vi "Filter_String_Parser.vi"(11 "Filter String":string="Protocol == UDP AND Length > 0.7 OR Source == 192.168.1.1") -> (1 "Comparators":T1(array[cluster]), 3 "Boolean Connectors":string[](array[string]))   [LabVIEW 2025, in "Table_Filtering.lvlib"]
uses:
  Table_Filtering.lvlib
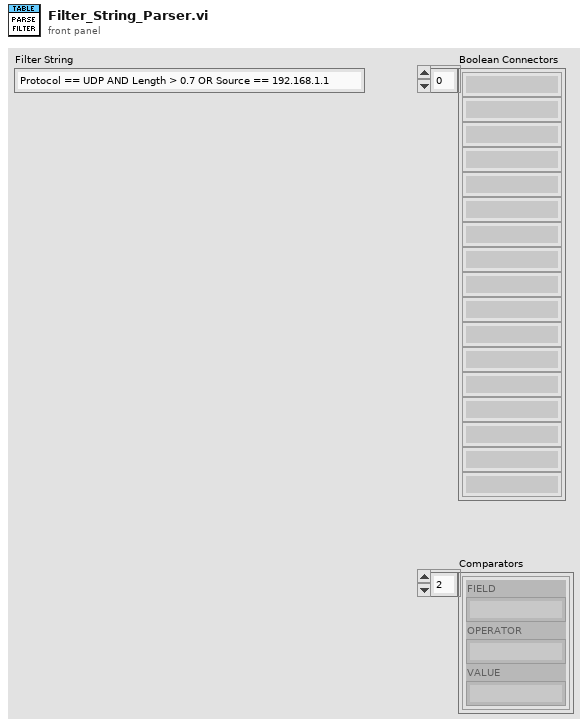
[diagram p1: front panel]
types:
  T1 = cluster{"FIELD":string, "OPERATOR":string, "VALUE":string}[]
  T2 = cluster{"FIELD":string, "OPERATOR":string, "VALUE":string}
  T3 = enum16{"Packet Number", "Timestamp", "Source", "Destination", "Protocol", "Length", "Data"}
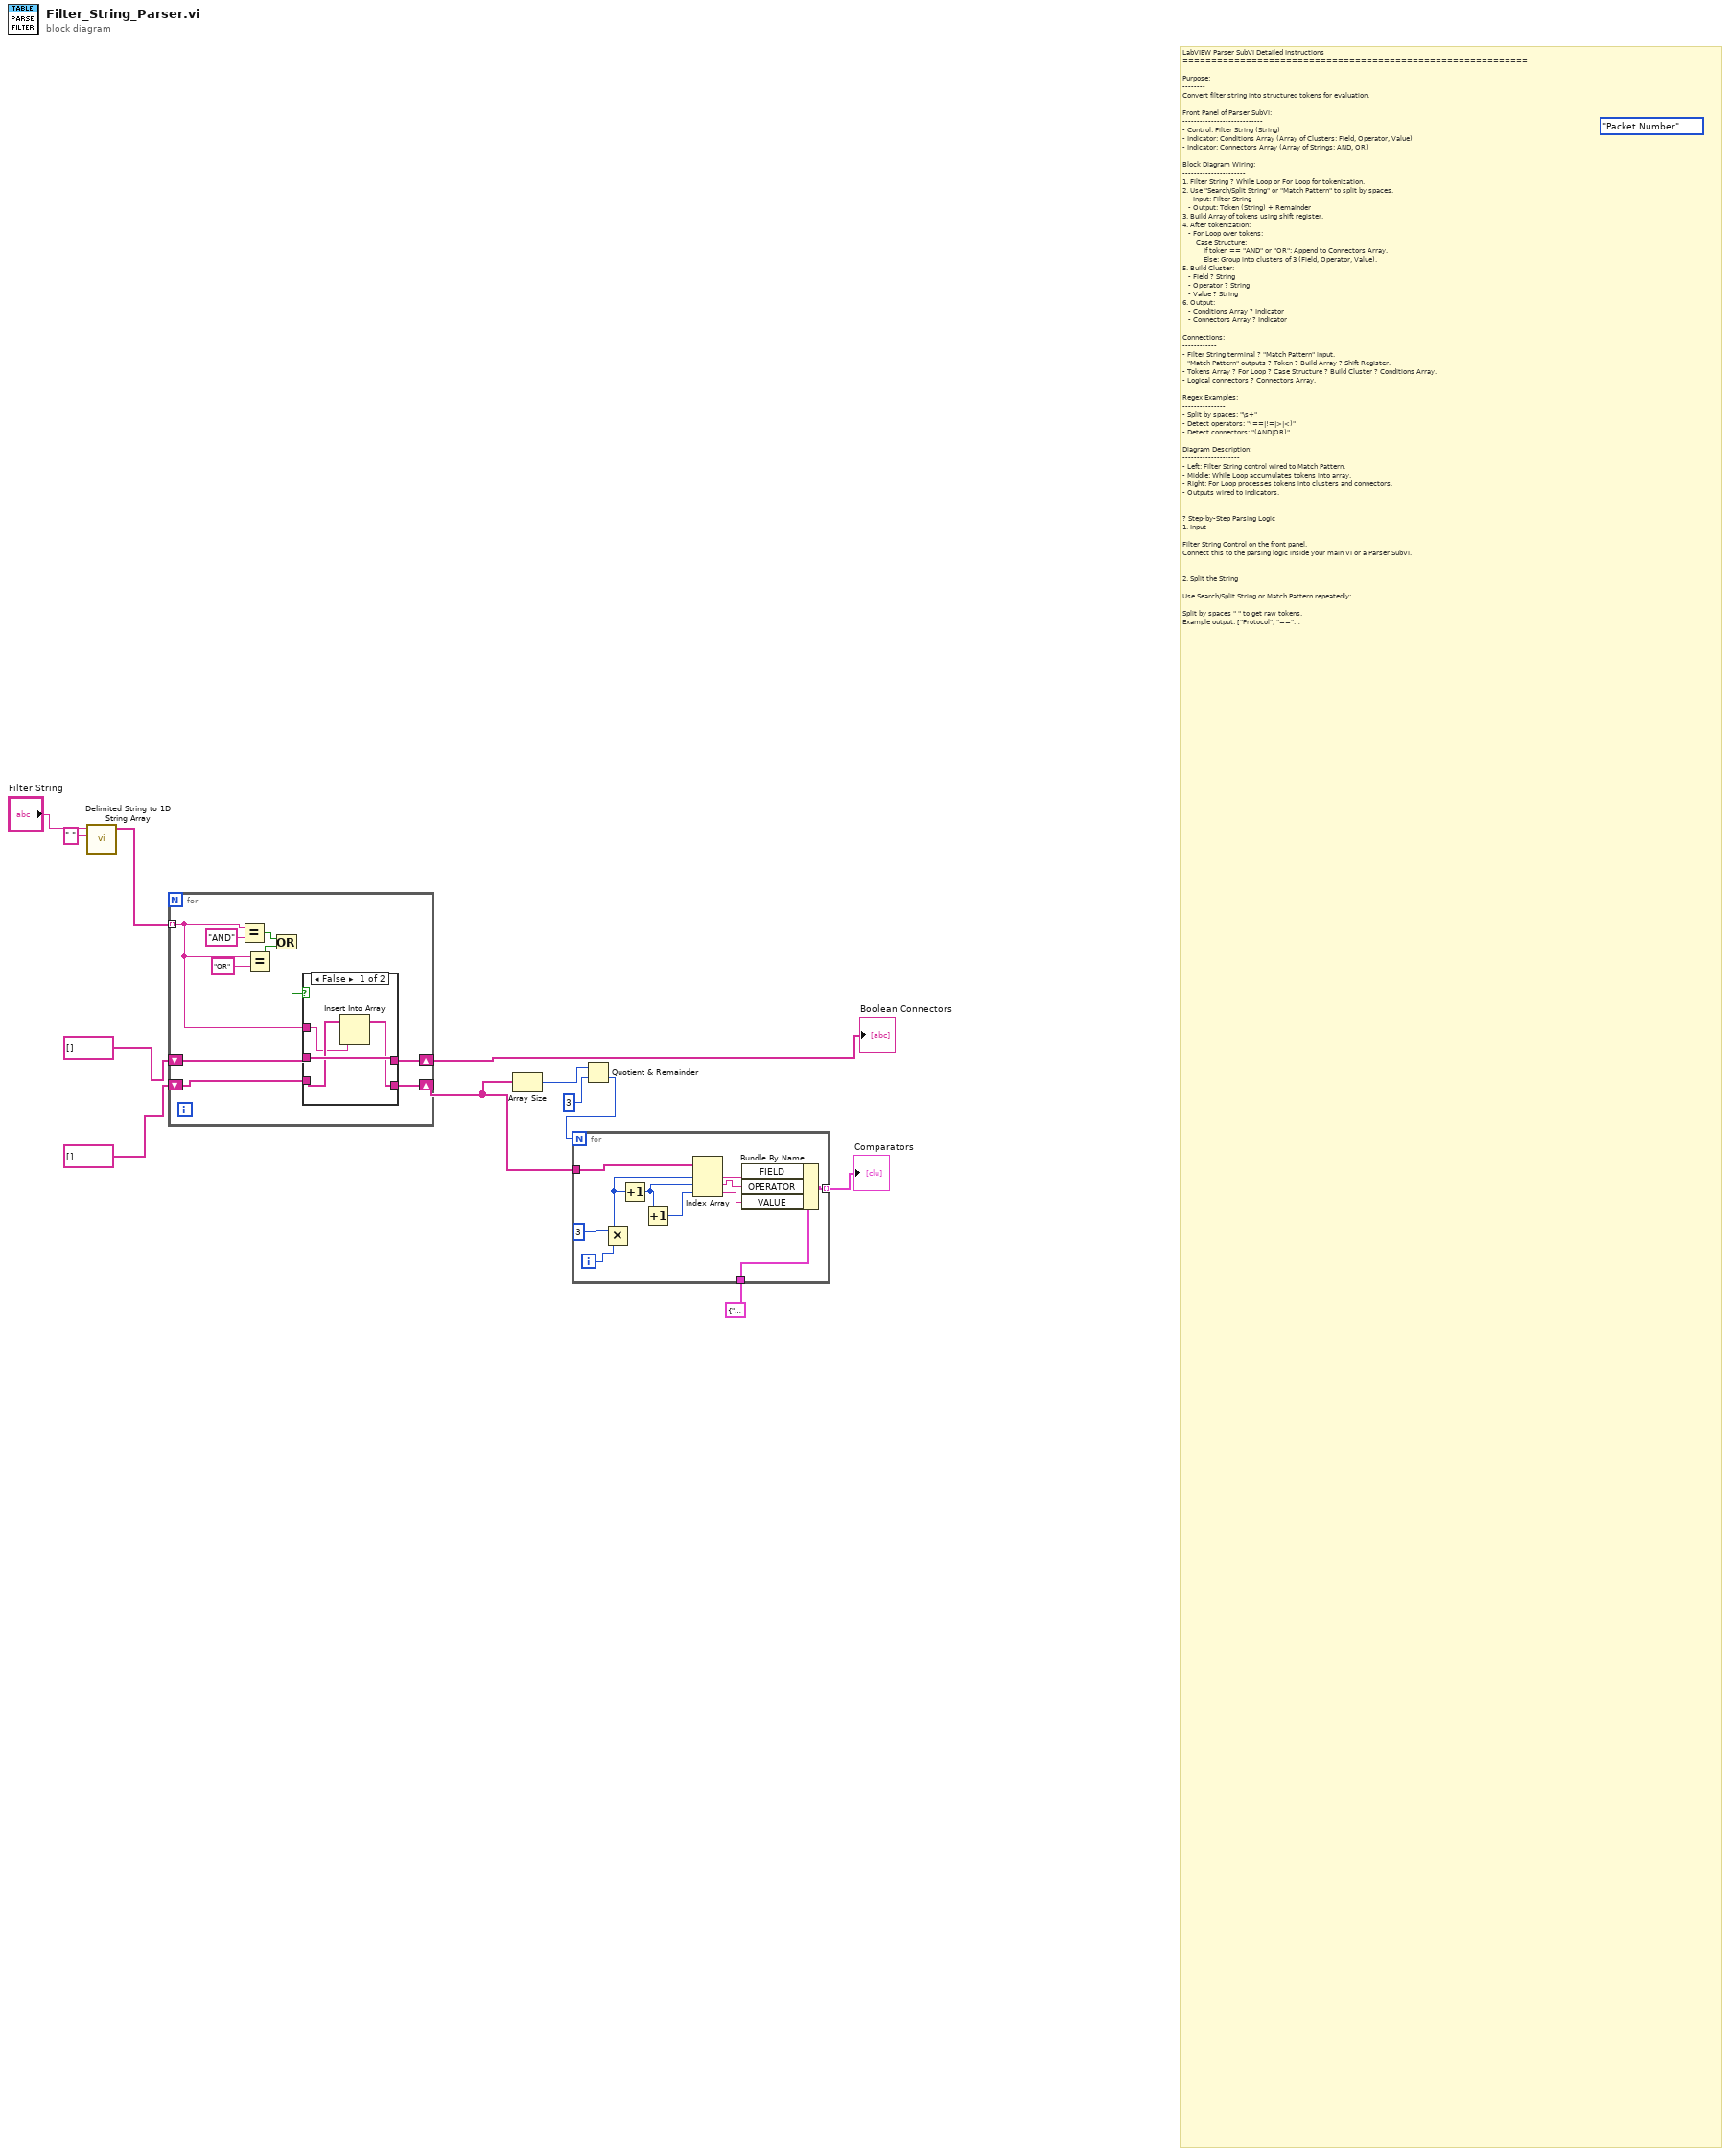
[diagram p0: block diagram]
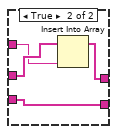
[diagram p2: hidden frame]
diagram:
  (unwired) T3."Packet Number" ("Sort By")
  # "LabVIEW Parser SubVI Detailed Instructions\n============================================================\n\nPurpose:\n--------\nConvert filter string into structured tokens for evaluation.\n\nFront Panel of Parser SubVI:\n----------------------------\n- Control: Filter String (String)\n- Indicator: Conditions Array (Array of Clusters: Field, Operator, Value)\n- Indicator: Connectors Array (Array of Strings: AND, OR)\n\nBlock Diagram Wiring:\n----------------------\n1. Filter String ? While Loop or For Loop for tokenization.\n2. Use \"Search/Split String\" or \"Match Pattern\" to split by spaces.\n   - Input: Filter String\n   - Output: Token (String) + Remainder\n3. Build Array of tokens using shift register.\n4. After tokenization:\n   - For Loop over tokens:\n       Case Structure:\n           If token == \"AND\" or \"OR\": Append to Connectors Array.\n           Else: Group into clusters of 3 (Field, Operator, Value).\n5. Build Cluster:\n   - Field ? String\n   - Operator ? String\n   - Value ? String\n6. Output:\n   - Conditions Array ? Indicator\n   - Connectors Array ? Indicator\n\nConnections:\n------------\n- Filter String terminal ? \"Match Pattern\" input.\n- \"Match Pattern\" outputs ? Token ? Build Array ? Shift Register.\n- Tokens Array ? For Loop ? Case Structure ? Build Cluster ? Conditions Array.\n- Logical connectors ? Connectors Array.\n\nRegex Examples:\n---------------\n- Split by spaces: \"\\s+\"\n- Detect operators: \"(==|!=|>|<)\"\n- Detect connectors: \"(AND|OR)\"\n\nDiagram Description:\n--------------------\n- Left: Filter String control wired to Match Pattern.\n- Middle: While Loop accumulates tokens into array.\n- Right: For Loop processes tokens into clusters and connectors.\n- Outputs wired to indicators.\n\n\n? Step-by-Step Parsing Logic\n1. Input\n\nFilter String Control on the front panel.\nConnect this to the parsing logic inside your main VI or a Parser SubVI.\n\n\n2. Split the String\n\nUse Search/Split String or Match Pattern repeatedly:\n\nSplit by spaces \" \" to get raw tokens.\nExample output: [\"Protocol\", \"==\", \"TCP\", \"AND\", \"Length\", \">\", \"100\", \"OR\", \"Source\", \"!=\", \"192.168.1.1\"].\n\n\n\nConnections:\n\nFilter String ? Search/Split String ? Array of Tokens.\n\n\n3. Identify Logical Connectors\n\nLoop through tokens:\n\nIf token = \"AND\" or \"OR\", mark as connector.\nElse, group into [Field, Operator, Value].\n\n\n\nConnections:\n\nArray of Tokens ? For Loop ? Case Structure:\n\nCase 1: Token is \"AND\" or \"OR\" ? Append to connector array.\nCase 2: Otherwise ? Append to condition array.\n\n\n\n\n4. Build Condition Clusters\n\nFor each [Field, Operator, Value] group:\n\nCreate a Cluster with:\n\nField (String)\nOperator (String)\nValue (String)\n\n\n\n\nStore connectors separately in an array.\n\nConnections:\n\nCondition Array ? Build Cluster ? Array of Clusters.\nConnector Array ? Array of Strings.\n\n\n5. Output\n\nTwo arrays:\n\nConditions Array (clusters of Field, Operator, Value)\nConnectors Array (strings: AND, OR)\n\n\n\nConnect these outputs to the Boolean Evaluation SubVI.\n\n? Boolean Evaluation SubVI Connections\n\nConditions Array ? For Loop:\n\nInside loop:\n\nExtract Field, Operator, Value.\nGet actual value from the current data row using Unbundle by Name.\nCompare using Case Structure for operator.\n\n\n\n\nConnectors Array ? Controls Boolean Combination:\n\nUse shift register to accumulate result:\n\nIf connector = AND ? result = result AND conditionResult\nIf connector = OR ? result = result OR conditionResult."
  n1 = call <vilib>:"Delimited String to 1D String Array.vi"("delimiter"=" ", "delimited string"="Filter String") -> ("string array"=w10:string[])  [unwired: 9 in]
  n2 = for {
    tunnel: w10 -> [w17] mode=indexing
    shift-right: [w13] -> w4
    shift-left: string[] [] -> [w16]
    shift-right: [w14] -> w3
    shift-left: string[] [] -> [w15]
    n3 = Equal?(x=w17, y="AND") -> (x = y?=w22:bool)
    n4 = Equal?(x=w17, y="OR") -> (x = y?=w19:bool)
    n5 = Or(x=w22, y=w19) -> (x .or. y?=w18:bool)
    n6 = case shown="False" w18 {
      tunnel: w17 -> [w24 w28]
      tunnel: w16 -> [w26 w29]
      tunnel: [w26 w27] -> w13
      tunnel: w15 -> [w25 w30]
      tunnel: [w23 w30] -> w14
      frame False {
        n7 = Insert Into Array(array=w25, new element=w24) -> (w23:string[])  [unwired: 1 in]
      }
      frame True {
        n8 = Insert Into Array(array=w29, new element=w28) -> (w27:string[])  [unwired: 1 in]
      }
    }
  }
  "Boolean Connectors" <- w4
  n9 = Array Size(array=w3) -> (size(s)=w8:i32)
  n10 = Quotient & Remainder(x=w8, y=3) -> (floor(x/y)=w1:i32)  [unwired: 1 out]
  n11 = for {
    N: w1 -> [_]
    tunnel: w3 -> [w41]
    tunnel: T2 {"FIELD"="", "OPERATOR"="", "VALUE"=""} -> [w35]
    tunnel: [w31] -> w6 mode=indexing
    i -> [w40]
    n12 = Multiply(x=3, y=w40) -> (x*y=w38:i32)
    n13 = Increment(x=w38) -> (x+1=w36:i32)
    n14 = Increment(x=w36) -> (x+1=w37:i32)
    n15 = Index Array(array=w41, index #1=w38, index #2=w36, index #3=w37) -> (element #1=w34:string, element #2=w33:string, element #3=w32:string)
    n16 = Bundle By Name(cluster=w35, "FIELD"=w34, "OPERATOR"=w33, "VALUE"=w32) -> (w31:T2)
  }
  "Comparators" <- w6
